vi "globalTearDown.vi"(8 "error in":errorcluster, 11 "Single Core Acyclic Loopback in":refnum<class "Single Core Acyclic Loopback.lvclass">) -> (0 "error out":errorcluster, 3 "Single Core Acyclic Loopback out":refnum<class "Single Core Acyclic Loopback.lvclass">)   [LabVIEW 2020, in "Single Core Acyclic Loopback.lvclass"]
uses:
  Single Core Acyclic Loopback.lvclass
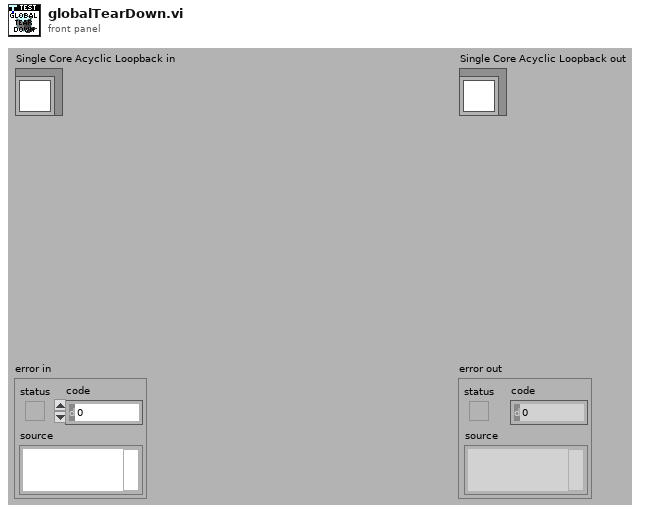
[diagram p1: front panel]
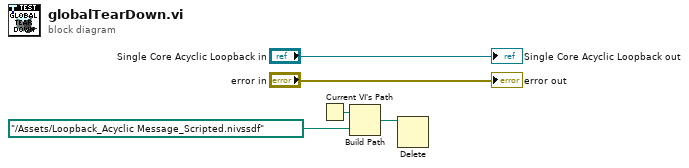
[diagram p0: block diagram]
diagram:
  n1 = Current VI's Path() -> (path=w2:path)
  n2 = Build Path(base path=w2, name or relative path=path "../Assets/Loopback_Acyclic Message_Scripted.nivssdf" ("Hardware File Path")) -> (appended path=w1:path)
  n3 = Delete(path (use dialog)=w1) -> ()  [unwired: 4 in, 3 out]
  "error out" <- "error in"
  "Single Core Acyclic Loopback out" <- "Single Core Acyclic Loopback in"
